vi "Clear.vi"(8 "error in (no error)":errorcluster, 11 "Graph Ref In":refnum<vi>) -> (0 "error out":errorcluster, 3 "Graph Ref Out":refnum<vi>)   [LabVIEW 2019, in "Graph Tools.lvlib"]
doc: "Clear Graph."
uses:
  Graph Tools.lvlib
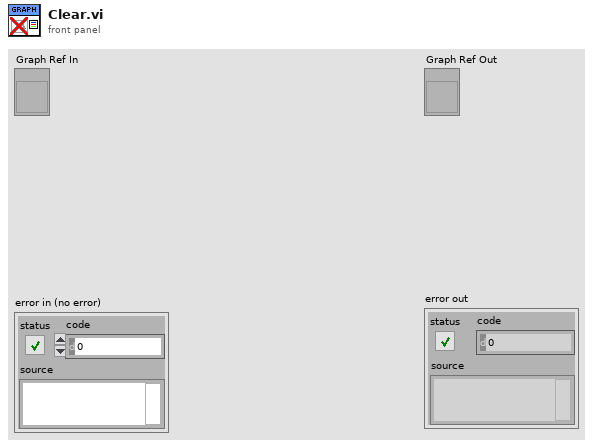
[diagram p1: front panel]
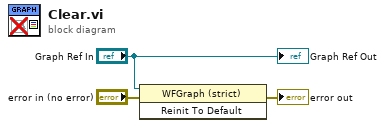
[diagram p0: block diagram]
diagram:
  n1 = invoke class="WFGraph (strict)" method="Reinit To Default"(reference="Graph Ref In", error in="error in (no error)") -> (error out=→"error out":errorcluster)  [unwired: 1 in, 2 out]
  "Graph Ref Out" <- "Graph Ref In"
